vi "SubVI Tester.vi"() -> ()   [LabVIEW 2012]
panel:
  in  "Min Temperature":dbl=10.0
  in  "Max Temperature":dbl=30.0
  in  "Stop":bool
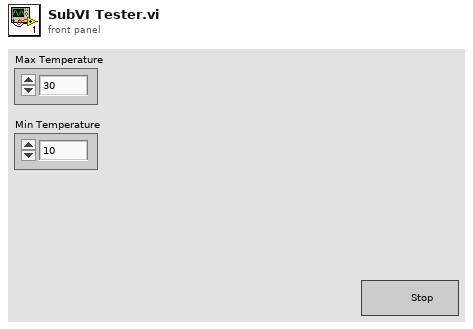
[diagram p1: front panel]
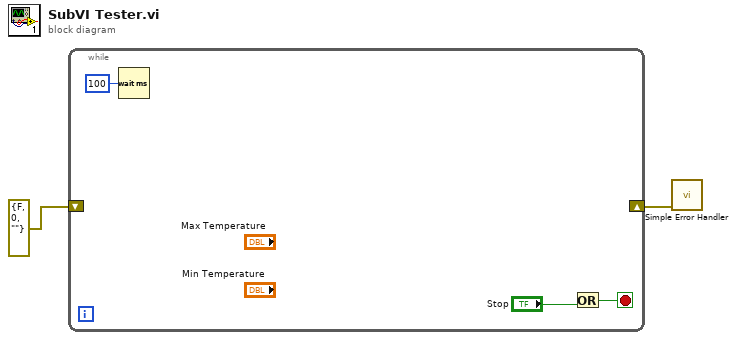
[diagram p0: block diagram]
diagram:
  n1 = while {
    shift-right: [_] -> w2
    shift-left: errorcluster {"status"=FALSE, "code"=0, "source"=""} ("error in") -> [_]
    stop <- w3 stop-if-true
    n2 = Wait (ms)(milliseconds to wait=u32 100) -> ()  [unwired: 1 out]
    n3 = Or(y="Stop") -> (x .or. y?=w3:bool)  [unwired: 1 in]
  }
  n4 = call <vilib>:"Simple Error Handler.vi"("error in (no error)"=w2) -> ()  [unwired: 4 in, 5 out]
